vi "Clear alarm signal.vi"(8 "error in (no error)":errorcluster, 11 "BoardHandle":T1) -> (0 "error out":errorcluster, 3 "BoardHandle out":T1)   [LabVIEW 2020, in "CAEN PSM.lvlib"]
doc: "Resets the status of alarms that occurred."
uses:
  CAEN PSM.lvlib
  Private/BoardHandle.ctl
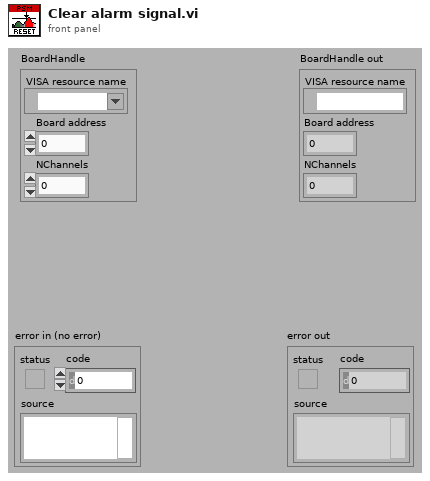
[diagram p1: front panel]
types:
  T1 = typedef "CAEN PSM.lvlib/BoardHandle.ctl" = cluster{"VISA resource name":refnum<visa-resource-name>, "Board address":i8, "NChannels":u8}
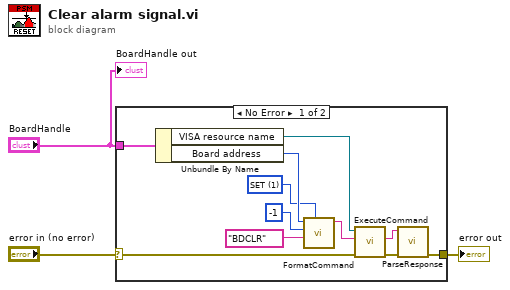
[diagram p0: block diagram]
diagram:
  n1 = case shown="No Error" "error in (no error)" {
    selector: "error in (no error)" -> [w6 w15]
    tunnel: [w9 w15] -> w2
    tunnel: "BoardHandle" -> [w7 _]
    frame No Error {
      w13 = u8 1 items=["MON", "SET"] ("CMD")
      n2 = Unbundle By Name(w7) -> ("VISA resource name"=w12:refnum<visa-resource-name>, "Board address"=w14:i8)
      n3 = call "FormatCommand.vi"("CMD (MON)"=w13, "PAR"="BDCLR", "CH"=i8 -1, "BD (0)"=w14) -> ("cmd"=w11:string)  [unwired: 7 in]
      n4 = call "ExecuteCommand.vi"("error in (no error)"=w6, "Command"=w11, "VISA resource name"=w12) -> ("error out"=w10:errorcluster, "Response"=w8:string)  [unwired: 6 in, 1 out]
      n5 = call "ParseResponse.vi"("error in (no error)"=w10, "Response"=w8) -> ("error out"=w9:errorcluster)  [unwired: 6 in, 3 out]
    }
    frame Error {
    }
  }
  "error out" <- w2
  "BoardHandle out" <- "BoardHandle"
